vi "progbar.vi"() -> ()   [LabVIEW 2011]
panel:
  out "Total Progress":dbl(slide) scale=0.0..1.0
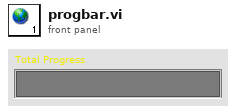
[diagram p1: front panel]
diagram:
